vi "trash_Node Status to gRPC Status to Manager.vi"(2 "Node Status":T21 {"Monitor Doubles"."4" format="%#_9g"; "Monitor Doubles"."3" format="%#_9g"; "Monitor Doubles"."2" format="%#_9g"; "Monitor Doubles"."1" format="%#_9g"; "Timing Statistics (us)"."Period"."Avg" format="%_6g"}) -> (4 "gRPC Status":T12)   [LabVIEW 2021]
uses:
  CIFCore/Grpc/CIFCorePlugin_client/RPC Messages/cif_plugincore_StatusData_State.ctl
  CIFCore/Grpc/CIFCorePlugin_client/CIFCorePlugin_client.lvlib
  CIFCore/Grpc/CIFCorePlugin_client/RPC Messages/cif_common_TimingStats.ctl
  CIFCore/Grpc/CIFCorePlugin_client/RPC Messages/cif_plugincore_TimingStatistics.ctl
  CIFCore/Grpc/CIFCorePlugin_client/RPC Messages/cif_plugincore_FifoStatistics.ctl
  CIFCore/Grpc/CIFCorePlugin_client/RPC Messages/cif_plugincore_Error.ctl
  CIFCore/Grpc/CIFCorePlugin_client/RPC Messages/cif_plugincore_MonitorDoubles.ctl
  CIFCore/Grpc/CIFCorePlugin_client/RPC Messages/cif_plugincore_MonitorU64.ctl
  CIFCore/Grpc/CIFCorePlugin_client/RPC Messages/cif_plugincore_MonitorI64.ctl
  CIFCore/Grpc/CIFCorePlugin_client/RPC Messages/cif_plugincore_StatusData.ctl
  CIFCore/Common/CIFCoreCommon.lvlib
  CIFCore/Common/Typedef/Simple Error.ctl
  CIFCore/Common/Typedef/Plugin State.ctl
  CIFCore/Common/Typedef/Plugin Status.ctl
  CIFCore/Common/Typedef/Timing Stats Base.ctl
  CIFCore/Common/Typedef/Timing Statistics.ctl
  CIFCore/Common/Typedef/FIFO Statistics.ctl
  CIFCore/Common/Typedef/Monitor Doubles.ctl
  CIFCore/Common/Typedef/Monitor U64.ctl
  CIFCore/Common/Typedef/Monitor I64.ctl
  CIF_Manager_client/RPC Messages/cif_plugincore_MonitorI64.ctl
  CIF_Manager_client/CIF_Manager_client.lvlib
  CIF_Manager_client/RPC Messages/cif_plugincore_MonitorU64.ctl
  CIF_Manager_client/RPC Messages/cif_plugincore_MonitorDoubles.ctl
  CIF_Manager_client/RPC Messages/cif_plugincore_Error.ctl
  CIF_Manager_client/RPC Messages/cif_common_TimingStats.ctl
  CIF_Manager_client/RPC Messages/cif_plugincore_FifoStatistics.ctl
  CIF_Manager_client/RPC Messages/cif_plugincore_TimingStatistics.ctl
  CIF_Manager_client/RPC Messages/cif_plugincore_StatusData_State.ctl
  CIF_Manager_client/RPC Messages/cif_plugincore_StatusData.ctl
  CIF_Manager_client/RPC Messages/cif_manager_PluginName.ctl
  CIF_Manager_client/RPC Messages/cif_manager_PluginStatus.ctl
panel:
  out "status":T1
  out "Status to Manager":T10
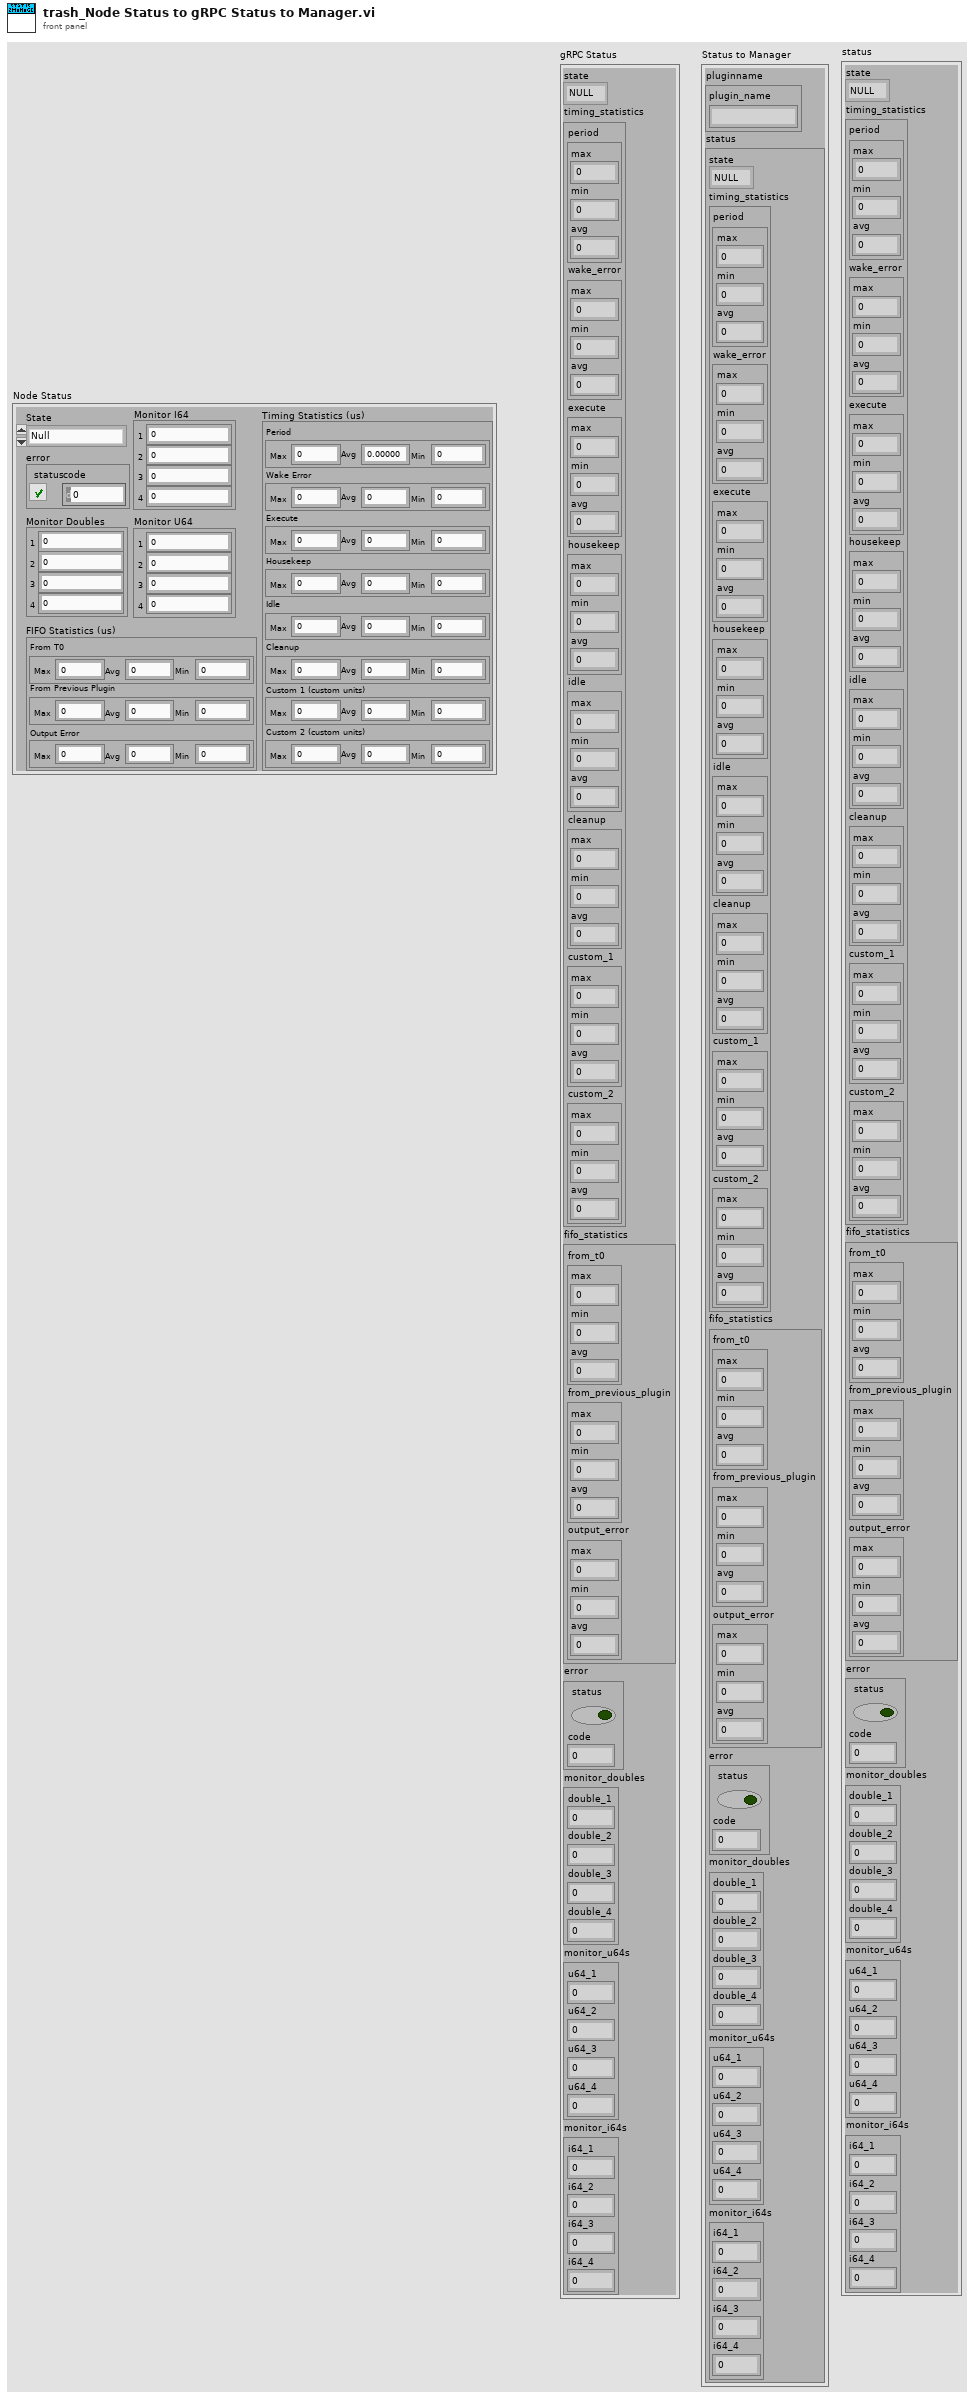
[diagram p1: front panel]
types:
  T1 = typedef "CIF_Manager_client.lvlib/cif_plugincore_StatusData.ctl" = cluster{"state":T2, "timing_statistics":T3, "fifo_statistics":T5, "error":T6, "monitor_doubles":T7, "monitor_u64s":T8, "monitor_i64s":T9}
  T2 = typedef "CIF_Manager_client.lvlib/cif_plugincore_StatusData_State.ctl" = enum32{"NULL", "CREATING", "LISTENING", "RUNNING", "CLEANINGUP", "DESTROYING"}
  T3 = typedef "CIF_Manager_client.lvlib/cif_plugincore_TimingStatistics.ctl" = cluster{"period":T4, "wake_error":T4, "execute":T4, "housekeep":T4, "idle":T4, "cleanup":T4, "custom_1":T4, "custom_2":T4}
  T4 = typedef "CIF_Manager_client.lvlib/cif_common_TimingStats.ctl" = cluster{"max":i64, "min":i64, "avg":dbl}
  T5 = typedef "CIF_Manager_client.lvlib/cif_plugincore_FifoStatistics.ctl" = cluster{"from_t0":T4, "from_previous_plugin":T4, "output_error":T4}
  T6 = typedef "CIF_Manager_client.lvlib/cif_plugincore_Error.ctl" = cluster{"status":bool, "code":i32}
  T7 = typedef "CIF_Manager_client.lvlib/cif_plugincore_MonitorDoubles.ctl" = cluster{"double_1":dbl, "double_2":dbl, "double_3":dbl, "double_4":dbl}
  T8 = typedef "CIF_Manager_client.lvlib/cif_plugincore_MonitorU64.ctl" = cluster{"u64_1":u64, "u64_2":u64, "u64_3":u64, "u64_4":u64}
  T9 = typedef "CIF_Manager_client.lvlib/cif_plugincore_MonitorI64.ctl" = cluster{"i64_1":i64, "i64_2":i64, "i64_3":i64, "i64_4":i64}
  T10 = typedef "CIF_Manager_client.lvlib/cif_manager_PluginStatus.ctl" = cluster{"pluginname":T11, "status":T1}
  T11 = typedef "CIF_Manager_client.lvlib/cif_manager_PluginName.ctl" = cluster{"plugin_name":string}
  T12 = typedef "CIFCorePlugin_client.lvlib/cif_plugincore_StatusData.ctl" = cluster{"state":T13, "timing_statistics":T14, "fifo_statistics":T16, "error":T17, "monitor_doubles":T18, "monitor_u64s":T19, "monitor_i64s":T20}
  T13 = typedef "CIFCorePlugin_client.lvlib/cif_plugincore_StatusData_State.ctl" = enum32{"NULL", "CREATING", "LISTENING", "RUNNING", "CLEANINGUP", "DESTROYING"}
  T14 = typedef "CIFCorePlugin_client.lvlib/cif_plugincore_TimingStatistics.ctl" = cluster{"period":T15, "wake_error":T15, "execute":T15, "housekeep":T15, "idle":T15, "cleanup":T15, "custom_1":T15, "custom_2":T15}
  T15 = typedef "CIFCorePlugin_client.lvlib/cif_common_TimingStats.ctl" = cluster{"max":i64, "min":i64, "avg":dbl}
  T16 = typedef "CIFCorePlugin_client.lvlib/cif_plugincore_FifoStatistics.ctl" = cluster{"from_t0":T15, "from_previous_plugin":T15, "output_error":T15}
  T17 = typedef "CIFCorePlugin_client.lvlib/cif_plugincore_Error.ctl" = cluster{"status":bool, "code":i32}
  T18 = typedef "CIFCorePlugin_client.lvlib/cif_plugincore_MonitorDoubles.ctl" = cluster{"double_1":dbl, "double_2":dbl, "double_3":dbl, "double_4":dbl}
  T19 = typedef "CIFCorePlugin_client.lvlib/cif_plugincore_MonitorU64.ctl" = cluster{"u64_1":u64, "u64_2":u64, "u64_3":u64, "u64_4":u64}
  T20 = typedef "CIFCorePlugin_client.lvlib/cif_plugincore_MonitorI64.ctl" = cluster{"i64_1":i64, "i64_2":i64, "i64_3":i64, "i64_4":i64}
  T21 = typedef "CIFCoreCommon.lvlib/Plugin Status.ctl" = cluster{"State":T22, "Timing Statistics (us)":T23, "FIFO Statistics (us)":T25, "error":T26, "Monitor Doubles":T27, "Monitor U64":T28, "Monitor I64":T29}
  T22 = typedef "CIFCoreCommon.lvlib/Plugin State.ctl" = enum32{"Null", "Creating", "Listening", "Running", "CleaningUp", "Destroying"}
  T23 = typedef "CIFCoreCommon.lvlib/Timing Statistics.ctl" = cluster{"Period":T24, "Wake Error":T24, "Execute":T24, "Housekeep":T24, "Idle":T24, "Cleanup":T24, "Custom 1 (custom units)":T24, "Custom 2 (custom units)":T24}
  T24 = typedef "CIFCoreCommon.lvlib/Timing Stats Base.ctl" = cluster{"Max":i64, "Avg":dbl, "Min":i64}
  T25 = typedef "CIFCoreCommon.lvlib/FIFO Statistics.ctl" = cluster{"From T0":T24, "From Previous Plugin":T24, "Output Error":T24}
  T26 = typedef "CIFCoreCommon.lvlib/Simple Error.ctl" = cluster{"status":bool, "code":i32}
  T27 = typedef "CIFCoreCommon.lvlib/Monitor Doubles.ctl" = cluster{"1":dbl, "2":dbl, "3":dbl, "4":dbl}
  T28 = typedef "CIFCoreCommon.lvlib/Monitor U64.ctl" = cluster{"1":u64, "2":u64, "3":u64, "4":u64}
  T29 = typedef "CIFCoreCommon.lvlib/Monitor I64.ctl" = cluster{"1":i64, "2":i64, "3":i64, "4":i64}
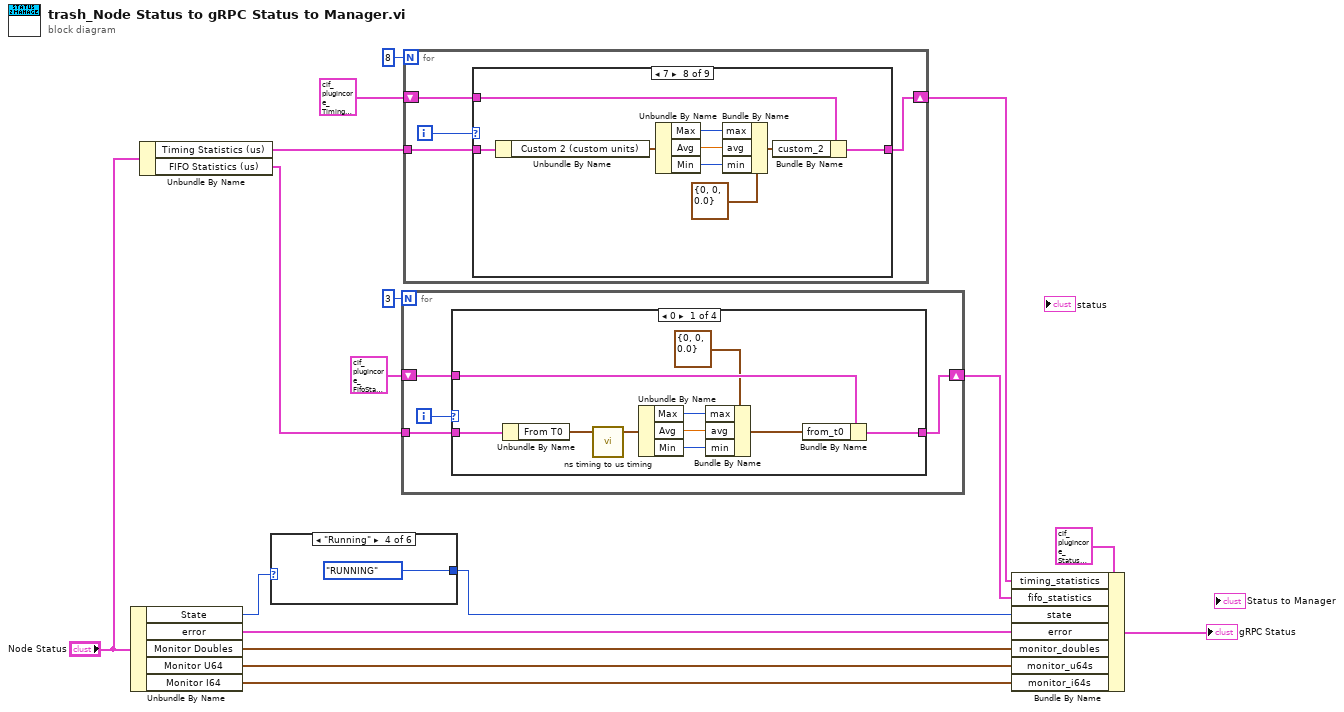
[diagram p0: block diagram]
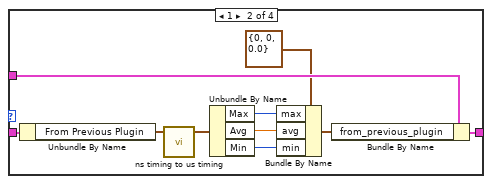
[diagram p2: hidden frame]
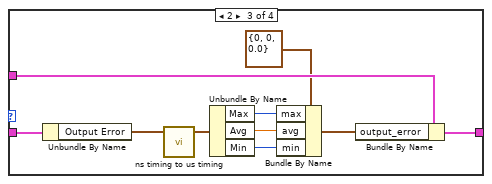
[diagram p3: hidden frame]
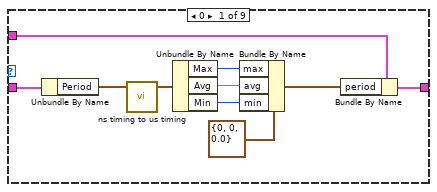
[diagram p5: hidden frame]
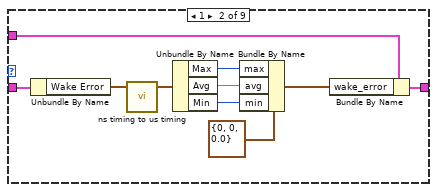
[diagram p6: hidden frame]
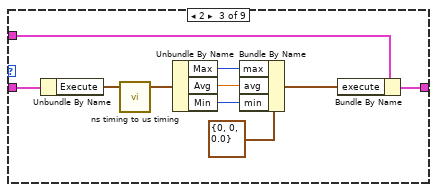
[diagram p7: hidden frame]
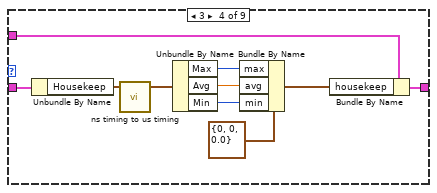
[diagram p8: hidden frame]
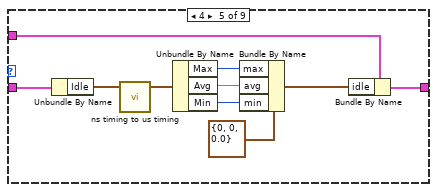
[diagram p9: hidden frame]
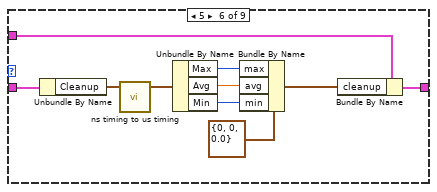
[diagram p10: hidden frame]
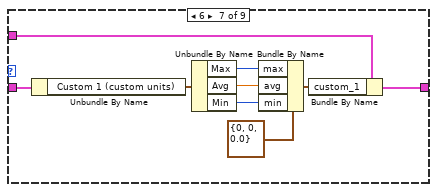
[diagram p11: hidden frame]
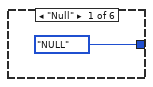
[diagram p13: hidden frame]
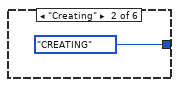
[diagram p14: hidden frame]
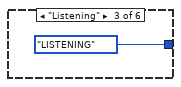
[diagram p15: hidden frame]
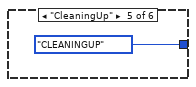
[diagram p16: hidden frame]
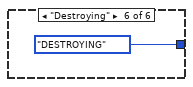
[diagram p17: hidden frame]
diagram:
  n1 = Unbundle By Name("Node Status") -> ("State"=w17:T22, "error"=w16:T26, "Monitor Doubles"=w15:T27, "Monitor U64"=w14:T28, "Monitor I64"=w13:T29)
  n2 = Unbundle By Name("Node Status") -> ("Timing Statistics (us)"=w9:T23, "FIFO Statistics (us)"=w8:T25)
  n3 = case shown="\"Running\"" w17 {
    tunnel: [cif_plugincore_StatusData_State."NULL" ("state") cif_plugincore_StatusData_State."CREATING" ("state") cif_plugincore_StatusData_State."LISTENING" ("state") cif_plugincore_StatusData_State."RUNNING" ("state") cif_plugincore_StatusData_State."CLEANINGUP" ("state") cif_plugincore_StatusData_State."DESTROYING" ("state")] -> w11
    frame "Null" {
    }
    frame "Creating" {
    }
    frame "Listening" {
    }
    frame "Running" {
    }
    frame "CleaningUp" {
    }
    frame "Destroying" {
    }
  }
  n4 = for {
    N: 3 -> [_]
    tunnel: w8 -> [w26]
    shift-right: [w25] -> w5
    shift-left: T16 {"from_t0"={"max"=0, "min"=0, "avg"=0.0}, "from_previous_plugin"={"max"=0, "min"=0, "avg"=0.0}, "output_error"={"max"=0, "min"=0, "avg"=0.0}} ("fifo_statistics") -> [w24]
    i -> [w27]
    n5 = case shown="0" w27 {
      tunnel: w26 -> [w31 w41 w51 _]
      tunnel: [w30 w40 w50 w58] -> w25
      tunnel: w24 -> [w29 w39 w49 w58]
      frame 0 {
        n6 = Unbundle By Name(w31) -> ("From T0"=w32:T24)
        n7 = call "ns timing to us timing.vi"("ns timing in"=w32) -> ("us timing out"=w37:T24)  [unwired: 4 in]
        n8 = Unbundle By Name(w37) -> ("Max"=w36:i64, "Avg"=w35:dbl, "Min"=w34:i64)
        n9 = Bundle By Name(cluster=T15 {"max"=0, "min"=0, "avg"=0.0} ("cif_plugincore_TimingStatsBasic"), "max"=w36, "avg"=w35, "min"=w34) -> (w33:T15)
        n10 = Bundle By Name(cluster=w29, "from_t0"=w33) -> (w30:T16)
      }
      frame 1 {
        n11 = Unbundle By Name(w41) -> ("From Previous Plugin"=w42:T24)
        n12 = call "ns timing to us timing.vi"("ns timing in"=w42) -> ("us timing out"=w47:T24)  [unwired: 4 in]
        n13 = Unbundle By Name(w47) -> ("Max"=w46:i64, "Avg"=w45:dbl, "Min"=w44:i64)
        n14 = Bundle By Name(cluster=T15 {"max"=0, "min"=0, "avg"=0.0} ("cif_plugincore_TimingStatsBasic"), "max"=w46, "avg"=w45, "min"=w44) -> (w43:T15)
        n15 = Bundle By Name(cluster=w39, "from_previous_plugin"=w43) -> (w40:T16)
      }
      frame 2 {
        n16 = Unbundle By Name(w51) -> ("Output Error"=w52:T24)
        n17 = call "ns timing to us timing.vi"("ns timing in"=w52) -> ("us timing out"=w57:T24)  [unwired: 4 in]
        n18 = Unbundle By Name(w57) -> ("Max"=w56:i64, "Avg"=w55:dbl, "Min"=w54:i64)
        n19 = Bundle By Name(cluster=T15 {"max"=0, "min"=0, "avg"=0.0} ("cif_plugincore_TimingStatsBasic"), "max"=w56, "avg"=w55, "min"=w54) -> (w53:T15)
        n20 = Bundle By Name(cluster=w49, "output_error"=w53) -> (w50:T16)
      }
      frame -1, Default {
      }
    }
  }
  n21 = for {
    N: 8 -> [_]
    tunnel: w9 -> [w61]
    shift-right: [w60] -> w4
    shift-left: T14 {"period"={"max"=0, "min"=0, "avg"=0.0}, "wake_error"={"max"=0, "min"=0, "avg"=0.0}, "execute"={"max"=0, "min"=0, "avg"=0.0}, "housekeep"={"max"=0, "min"=0, "avg"=0.0}, "idle"={"max"=0, "min"=0, "avg"=0.0}, "cleanup"={"max"=0, "min"=0, "avg"=0.0}, "custom_1"={"max"=0, "min"=0, "avg"=0.0}, "custom_2"={"max"=0, "min"=0, "avg"=0.0}} ("timing_statistics") -> [w59]
    i -> [w62]
    n22 = case shown="7" w62 {
      tunnel: w61 -> [w64 w74 w91 w101 w111 w121 w131 w140 _]
      tunnel: [w72 w82 w90 w100 w110 w120 w130 w139 w141] -> w60
      tunnel: w59 -> [w71 w81 w89 w99 w109 w119 w129 w138 w141]
      frame 0 {
        n23 = Unbundle By Name(w64) -> ("Period"=w63:T24)
        n24 = call "ns timing to us timing.vi"("ns timing in"=w63) -> ("us timing out"=w70:T24)  [unwired: 4 in]
        n25 = Unbundle By Name(w70) -> ("Max"=w68:i64, "Avg"=w67:dbl, "Min"=w66:i64)
        n26 = Bundle By Name(cluster=T15 {"max"=0, "min"=0, "avg"=0.0} ("timing_statistics.period"), "max"=w68, "avg"=w67, "min"=w66) -> (w65:T15)
        n27 = Bundle By Name(cluster=w71, "period"=w65) -> (w72:T14)
      }
      frame 1 {
        n28 = Unbundle By Name(w74) -> ("Wake Error"=w73:T24)
        n29 = call "ns timing to us timing.vi"("ns timing in"=w73) -> ("us timing out"=w80:T24)  [unwired: 4 in]
        n30 = Unbundle By Name(w80) -> ("Max"=w78:i64, "Avg"=w77:dbl, "Min"=w76:i64)
        n31 = Bundle By Name(cluster=T15 {"max"=0, "min"=0, "avg"=0.0} ("timing_statistics.period"), "max"=w78, "avg"=w77, "min"=w76) -> (w75:T15)
        n32 = Bundle By Name(cluster=w81, "wake_error"=w75) -> (w82:T14)
      }
      frame 2 {
        n33 = Unbundle By Name(w91) -> ("Execute"=w92:T24)
        n34 = call "ns timing to us timing.vi"("ns timing in"=w92) -> ("us timing out"=w88:T24)  [unwired: 4 in]
        n35 = Unbundle By Name(w88) -> ("Max"=w86:i64, "Avg"=w85:dbl, "Min"=w84:i64)
        n36 = Bundle By Name(cluster=T15 {"max"=0, "min"=0, "avg"=0.0} ("timing_statistics.period"), "max"=w86, "avg"=w85, "min"=w84) -> (w83:T15)
        n37 = Bundle By Name(cluster=w89, "execute"=w83) -> (w90:T14)
      }
      frame 3 {
        n38 = Unbundle By Name(w101) -> ("Housekeep"=w102:T24)
        n39 = call "ns timing to us timing.vi"("ns timing in"=w102) -> ("us timing out"=w98:T24)  [unwired: 4 in]
        n40 = Unbundle By Name(w98) -> ("Max"=w97:i64, "Avg"=w96:dbl, "Min"=w95:i64)
        n41 = Bundle By Name(cluster=T15 {"max"=0, "min"=0, "avg"=0.0} ("cif_plugincore_TimingStatsBasic"), "max"=w97, "avg"=w96, "min"=w95) -> (w94:T15)
        n42 = Bundle By Name(cluster=w99, "housekeep"=w94) -> (w100:T14)
      }
      frame 4 {
        n43 = Unbundle By Name(w111) -> ("Idle"=w112:T24)
        n44 = call "ns timing to us timing.vi"("ns timing in"=w112) -> ("us timing out"=w108:T24)  [unwired: 4 in]
        n45 = Unbundle By Name(w108) -> ("Max"=w106:i64, "Avg"=w105:dbl, "Min"=w104:i64)
        n46 = Bundle By Name(cluster=T15 {"max"=0, "min"=0, "avg"=0.0} ("timing_statistics.period"), "max"=w106, "avg"=w105, "min"=w104) -> (w103:T15)
        n47 = Bundle By Name(cluster=w109, "idle"=w103) -> (w110:T14)
      }
      frame 5 {
        n48 = Unbundle By Name(w121) -> ("Cleanup"=w122:T24)
        n49 = call "ns timing to us timing.vi"("ns timing in"=w122) -> ("us timing out"=w118:T24)  [unwired: 4 in]
        n50 = Unbundle By Name(w118) -> ("Max"=w116:i64, "Avg"=w115:dbl, "Min"=w114:i64)
        n51 = Bundle By Name(cluster=T15 {"max"=0, "min"=0, "avg"=0.0} ("timing_statistics.period"), "max"=w116, "avg"=w115, "min"=w114) -> (w113:T15)
        n52 = Bundle By Name(cluster=w119, "cleanup"=w113) -> (w120:T14)
      }
      frame 6 {
        n53 = Unbundle By Name(w131) -> ("Custom 1 (custom units)"=w123:T24)
        n54 = Unbundle By Name(w123) -> ("Max"=w127:i64, "Avg"=w126:dbl, "Min"=w125:i64)
        n55 = Bundle By Name(cluster=T15 {"max"=0, "min"=0, "avg"=0.0} ("timing_statistics.period"), "max"=w127, "avg"=w126, "min"=w125) -> (w124:T15)
        n56 = Bundle By Name(cluster=w129, "custom_1"=w124) -> (w130:T14)
      }
      frame 7 {
        n57 = Unbundle By Name(w140) -> ("Custom 2 (custom units)"=w132:T24)
        n58 = Unbundle By Name(w132) -> ("Max"=w136:i64, "Avg"=w135:dbl, "Min"=w134:i64)
        n59 = Bundle By Name(cluster=T15 {"max"=0, "min"=0, "avg"=0.0} ("timing_statistics.period"), "max"=w136, "avg"=w135, "min"=w134) -> (w133:T15)
        n60 = Bundle By Name(cluster=w138, "custom_2"=w133) -> (w139:T14)
      }
      frame -1, Default {
      }
    }
  }
  n61 = Bundle By Name(cluster=T12 {"state"=enum."NULL", "timing_statistics"={"period"={"max"=0, "min"=0, "avg"=0.0}, "wake_error"={"max"=0, "min"=0, "avg"=0.0}, "execute"={"max"=0, "min"=0, "avg"=0.0}, "housekeep"={"max"=0, "min"=0, "avg"=0.0}, "idle"={"max"=0, "min"=0, "avg"=0.0}, "cleanup"={"max"=0, "min"=0, "avg"=0.0}, "custom_1"={"max"=0, "min"=0, "avg"=0.0}, "custom_2"={"max"=0, "min"=0, "avg"=0.0}}, "fifo_statistics"={"from_t0"={"max"=0, "min"=0, "avg"=0.0}, "from_previous_plugin"={"max"=0, "min"=0, "avg"=0.0}, "output_error"={"max"=0, "min"=0, "avg"=0.0}}, "error"={"status"=FALSE, "code"=0}, "monitor_doubles"={"double_1"=0.0, "double_2"=0.0, "double_3"=0.0, "double_4"=0.0}, "monitor_u64s"={"u64_1"=0, "u64_2"=0, "u64_3"=0, "u64_4"=0}, "monitor_i64s"={"i64_1"=0, "i64_2"=0, "i64_3"=0, "i64_4"=0}} ("gRPC Status"), "timing_statistics"=w4, "fifo_statistics"=w5, "state"=w11, "error"=w16, "monitor_doubles"=w15, "monitor_u64s"=w14, "monitor_i64s"=w13) -> (→"gRPC Status":T12)
